vi "Insert (element).vi"(8 "error in (no error)":errorcluster, 10 "Key-Value Pair":T1, 11 "Parameter to Hardware Map in":refnum<class "Parameter to Hardware Map.lvclass">) -> (0 "error out":errorcluster, 3 "Parameter to Hardware Map out":refnum<class "Parameter to Hardware Map.lvclass">)   [LabVIEW 2020, in "Parameter to Hardware Map.lvclass"]
doc: "Insert the given key-value pair into the map."
uses:
  Parameter to Hardware Map.lvclass
  Controller/Generic Plugin.lvclass
  Pair.ctl
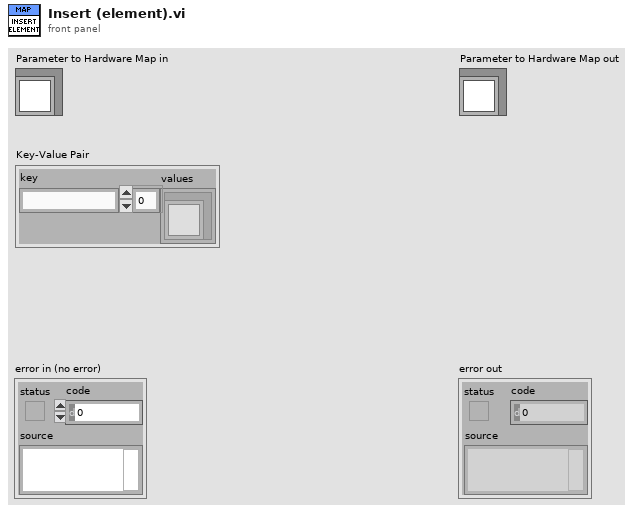
[diagram p1: front panel]
types:
  T1 = typedef "Parameter to Hardware Map.lvclass/Pair.ctl" = cluster{"key":string, "values":refnum<class "Generic Plugin.lvclass">[]}
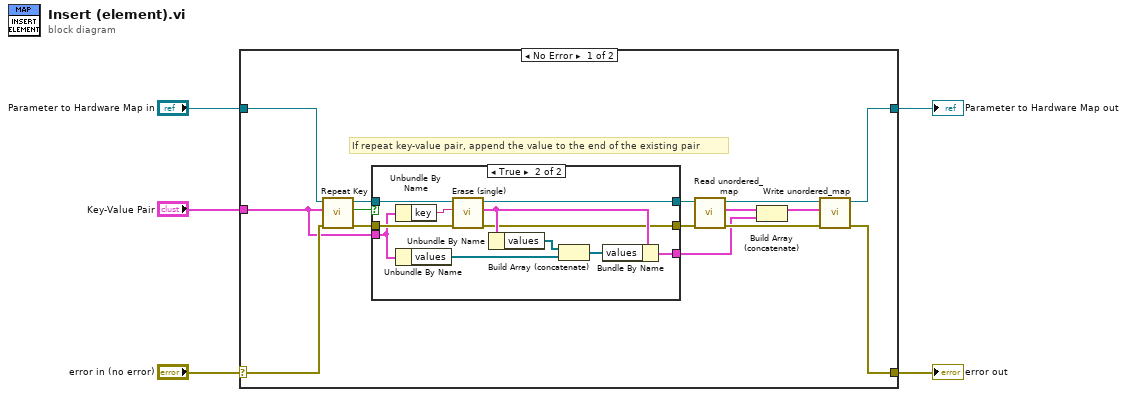
[diagram p0: block diagram]
diagram:
  n1 = case shown="No Error" "error in (no error)" {
    selector: "error in (no error)" -> [w19 w36]
    tunnel: [w8 w36] -> w4
    tunnel: [w7 w35] -> w2
    tunnel: "Parameter to Hardware Map in" -> [w20 w35]
    tunnel: "Key-Value Pair" -> [w16 _]
    frame No Error {
      # "If repeat key-value pair, append the value to the end of the existing pair"
      n2 = call "Repeat Key.vi"("error in (no error)"=w19, "Key-Value Pair"=w16, "Parameter to Hardware Map in"=w20) -> ("error out"=w18:errorcluster, "Repeat?"=w15:bool, "Parameter to Hardware Map out"=w17:refnum<class "Parameter to Hardware Map.lvclass">)  [unwired: 6 in]
      n3 = case shown="True" w15 {
        tunnel: w18 -> [w23 w31]
        tunnel: w17 -> [w22 w34]
        tunnel: w16 -> [w21 w30]
        tunnel: [w23 w24] -> w9
        tunnel: [w22 w33] -> w10
        tunnel: [w21 w25] -> w6
        frame False {
        }
        frame True {
          n4 = Unbundle By Name(w30) -> ("key"=w32:string)
          n5 = Unbundle By Name(w30) -> ("values"=w28:refnum<class "Generic Plugin.lvclass">[])
          n6 = call "Erase (single).vi"("error in (no error)"=w31, "Key"=w32, "Parameter to Hardware Map in"=w34) -> ("error out"=w24:errorcluster, "Deleted Pair"=w27:T1, "Parameter to Hardware Map out"=w33:refnum<class "Parameter to Hardware Map.lvclass">)  [unwired: 6 in]
          n7 = Unbundle By Name(w27) -> ("values"=w29:refnum<class "Generic Plugin.lvclass">[])
          n8 = Build Array (concatenate)(w29, w28) -> (w26:refnum<class "Generic Plugin.lvclass">[])
          n9 = Bundle By Name(cluster=w27, "values"=w26) -> (w25:T1)
        }
      }
      n10 = call "Read unordered_map.vi"("error in (no error)"=w9, "Parameter to Hardware Map in"=w10) -> ("error out"=w11:errorcluster, "unordered_map"=w12:T1[], "Parameter to Hardware Map out"=w13:refnum<class "Parameter to Hardware Map.lvclass">)  [unwired: 7 in]
      n11 = Build Array (concatenate)(w12, w6) -> (w14:T1[])
      n12 = call "Write unordered_map.vi"("error in (no error)"=w11, "unordered_map"=w14, "Parameter to Hardware Map in"=w13) -> ("error out"=w8:errorcluster, "Parameter to Hardware Map out"=w7:refnum<class "Parameter to Hardware Map.lvclass">)  [unwired: 7 in]
    }
    frame Error {
    }
  }
  "error out" <- w4
  "Parameter to Hardware Map out" <- w2
